vi "SimularOnda.vi"(0 "Sinal":string, 1 "Tempo":dbl min=0.0, 2 "Offset":dbl min=-10.0 max=10.0, 3 "Amplitude":dbl min=0.0 max=10.0, 4 "Fase":dbl, 5 "Frequencia":dbl, 6 "RazaoCiclica":dbl, 8 "LabVIEW Web Service Request":refnum<class "Web Request.lvclass">) -> ()   [LabVIEW 2020]
uses:
  <vilib>/wsapi/Web Request.lvclass
  5bb1ef98-1994-4d65-9c78-bc6588d51ed2.vi
panel:
  # "Use the Web Service Request input terminal to call the VIs on the Web Services palette. Do not remove it from the connector pane unless you don't need access to the palette."
  # "Each additional control wired to the connector pane will be available as an input in the URL. To include an indicator in terminal-mode output (the default setting), it must also be wired to the connector pane."
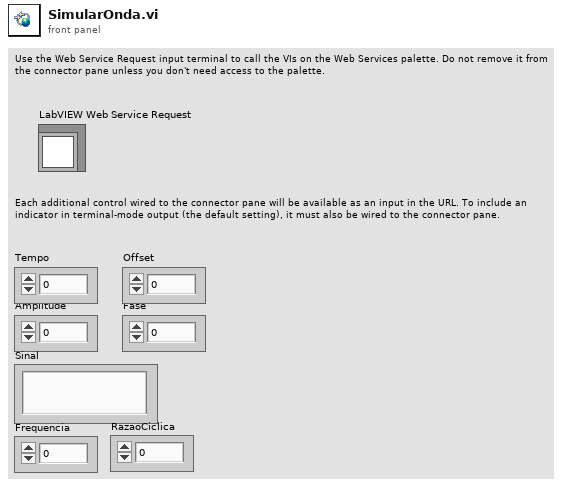
[diagram p1: front panel]
types:
  T1 = enum16{"create", "fire - Simular onda", "fire - Editar onda", "destroy"}
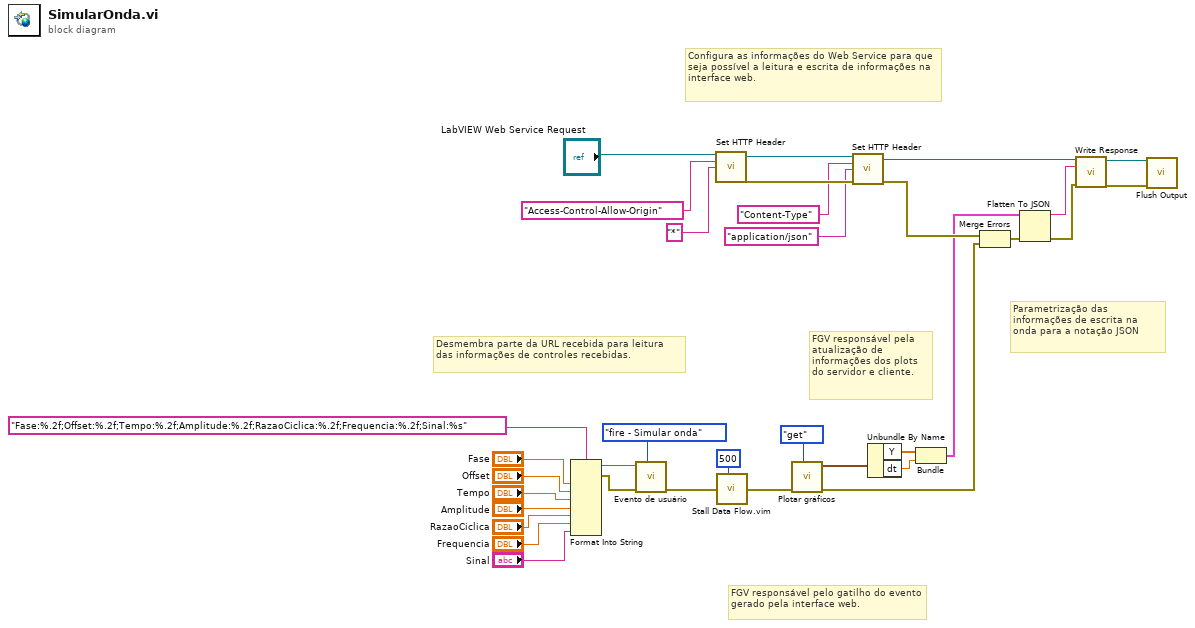
[diagram p0: block diagram]
diagram:
  # "Parametrização das informações de escrita na onda para a notação JSON"
  # "FGV responsável pela atualização de informações dos plots do servidor e cliente."
  # "FGV responsável pelo gatilho do evento gerado pela interface web."
  # "Desmembra parte da URL recebida para leitura das informações de controles recebidas."
  # "Configura as informações do Web Service para que seja possível a leitura e escrita de informações na interface web."
  n1 = Format Into String(format string="Fase:%.2f;Offset:%.2f;Tempo:%.2f;Amplitude:%.2f;RazaoCiclica:%.2f;Frequencia:%.2f;Sinal:%s", "Fase", "Offset", "Tempo", "Amplitude", "RazaoCiclica", "Frequencia", "Sinal") -> (resulting string=w18:string, error out=w14:errorcluster)  [unwired: 2 in]
  n2 = call "Evento de usuário.vi"("Enum"=T1."fire - Simular onda", "error in (no error)"=w14, "Dados"=w18) -> ("error out"=w17:errorcluster)  [unwired: 7 in, 1 out]
  n3 = call <vilib>:"Set HTTP Header.vi"("LabVIEW Web Service Request"="LabVIEW Web Service Request", "header"="Access-Control-Allow-Origin", "header value"="*") -> ("LabVIEW Web Service Request out"=w34:refnum<class "Web Request.lvclass">, "error out"=w33:errorcluster)  [unwired: 11 in]
  n4 = call "Stall Data Flow.vim"("value in"=w17, "milliseconds to wait"=u32 500) -> ("value out"=w16:errorcluster)  [unwired: 1 out]
  n5 = call "Plotar gráficos.vi"("Enum"=enum16{"set", "get"}."get", "error in (no error)"=w16) -> ("error out"=w12:errorcluster, "Plot"=w8:waveform(dbl))  [unwired: 8 in]
  n6 = call <vilib>:"Set HTTP Header.vi"("LabVIEW Web Service Request"=w34, "header"="Content-Type", "header value"="application/json", "error in (no error)"=w33) -> ("LabVIEW Web Service Request out"=w32:refnum<class "Web Request.lvclass">, "error out"=w11:errorcluster)  [unwired: 10 in]
  n7 = Unbundle By Name(w8) -> ("Y"=w10:dbl[], "dt"=w9:dbl)
  n8 = Bundle("Y"=w10, "dt"=w9) -> (w7:cluster{"Y":dbl[], "dt":dbl})  [unwired: 1 in]
  n9 = Merge Errors(w11, w12) -> (w13:errorcluster)
  n10 = Flatten To JSON(anything=w7, error in (no error)=w13) -> (JSON string=w24:string, 11:w1:errorcluster)  [unwired: 1 in]
  n11 = call <vilib>:"Write Response.vi"("LabVIEW Web Service Request"=w32, "response string"=w24, "error in (no error)"=w1) -> ("LabVIEW Web Service Request out"=w26:refnum<class "Web Request.lvclass">, "error out"=w25:errorcluster)  [unwired: 11 in]
  n12 = call <vilib>:"Flush Output.vi"("LabVIEW Web Service Request"=w26, "error in (no error)"=w25) -> ()  [unwired: 12 in, 2 out]
